vi "Increment Progress.vi"(11 "Execution UI In":refnum<class "Execution UI.lvclass">) -> (2 "Progress (%)":dbl, 3 "Execution UI Out":refnum<class "Execution UI.lvclass">)   [LabVIEW 2020, in "Execution UI.lvclass"]
uses:
  Execution UI.lvclass
  Test Suite/LUnit Test Suite.lvclass
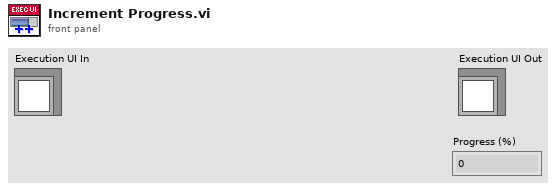
[diagram p1: front panel]
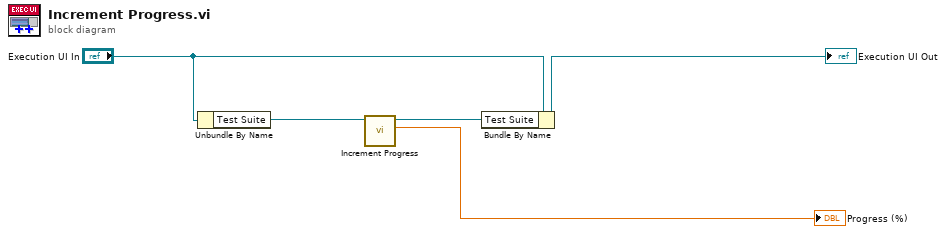
[diagram p0: block diagram]
diagram:
  n1 = Unbundle By Name("Execution UI In") -> ("Test Suite"=w4:refnum<class "LUnit Test Suite.lvclass">)
  n2 = call "Increment Progress.vi"("LUnit Test Suite in"=w4) -> ("Progress (%)"=→"Progress (%)":dbl, "LUnit Test Suite out"=w2:refnum<class "LUnit Test Suite.lvclass">)  [unwired: 9 in]
  n3 = Bundle By Name(cluster="Execution UI In", "Test Suite"=w2) -> (→"Execution UI Out":refnum<class "Execution UI.lvclass">)
